vi "Initialize SCIP2.vi"(8 "error in (no error)":errorcluster, 11 "VISA Refnum in":refnum<visa-resource-name>) -> (0 "error out":errorcluster, 3 "VISA Refnum out":refnum<visa-resource-name>)   [LabVIEW 2016]
doc: "Set the URG-04LX to use the SCIP2.0 protocol."
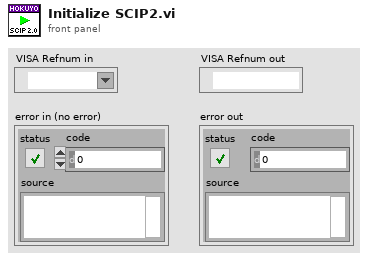
[diagram p1: front panel]
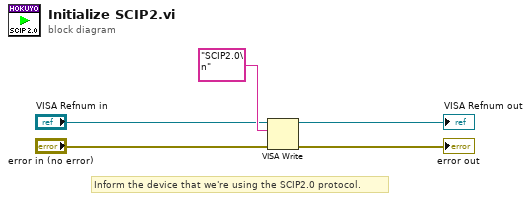
[diagram p0: block diagram]
diagram:
  # "Inform the device that we're using the SCIP2.0 protocol."
  n1 = VISA Write(VISA resource name="VISA Refnum in", write buffer="SCIP2.0\n", error in (no error)="error in (no error)") -> (VISA resource name out=→"VISA Refnum out":refnum<visa-resource-name>, error out=→"error out":errorcluster)  [unwired: 1 out]
